vi "limit string size.vi"(0 "string in":string, 1 "byte limit (1MB)":i32=1048576) -> (2 "string out":string)   [LabVIEW 2024, in "status manager.lvlib"]
uses:
  status manager.lvlib
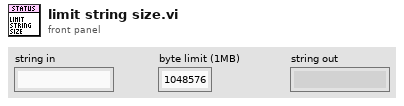
[diagram p1: front panel]
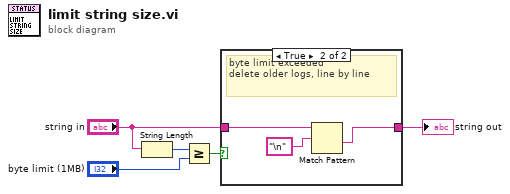
[diagram p0: block diagram]
diagram:
  n1 = String Length(string="string in") -> (length=w1:i32)
  n2 = Greater Or Equal?(x=w1, y="byte limit (1MB)") -> (x >= y?=w3:bool)
  n3 = case shown="True" w3 {
    tunnel: "string in" -> [w6 w9]
    tunnel: [w6 w7] -> w4
    frame False {
      # "byte limit not exceeded\ndo nothing"
    }
    frame True {
      # "byte limit exceeded\ndelete older logs, line by line"
      n4 = Match Pattern(string=w9, regular expression="\n") -> (after substring=w7:string)  [unwired: 1 in, 3 out]
    }
  }
  "string out" <- w4
